vi "DataSocket-ImgSender.vi"() -> ()   [LabVIEW 2019]
doc: "Uses DataSocket to write array data. This example works for writing the data to the DataSocket Server (for live data). \n \nThe Writer, Server, and Reader can all be on the same computer or different computers. The Writer and Reader URLs should point to the computer where the DataSocket Server is."
panel:
  out "Image":T1(plugin-control)
  in  "Stop":bool
  # "DataSocket - Image Sender"
  # "Instruction:\n1. Run DataSocket Server;\n2. Run this VI;\n3. Run Image Receiver.\n4. see the images transfered\n to image reveiver."
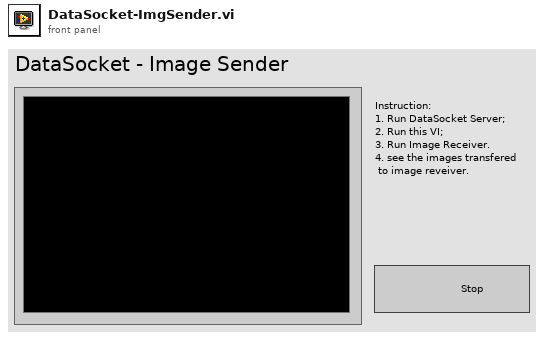
[diagram p1: front panel]
types:
  T1 = typedef "IMAQ Image.ctl" = refnum<image>
  T2 = enum16{"Read", "Write", "ReadWrite", "BufferedRead", "BufferedReadWrite"}
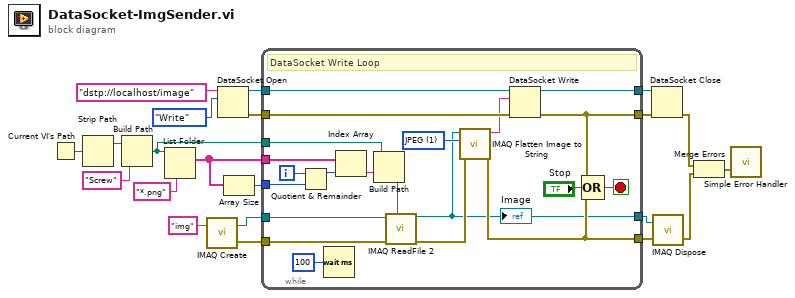
[diagram p0: block diagram]
diagram:
  n1 = Current VI's Path() -> (path=w12:path)
  n2 = Strip Path(path=w12) -> (stripped path=w11:path)  [unwired: 1 out]
  n3 = Build Path(base path=w11, name or relative path="Screw") -> (appended path=w6:path)
  n4 = List Folder(path=w6, pattern="*.png") -> (filenames=w4:string[])  [unwired: 2 in, 3 out]
  n5 = call "IMAQ Create"("Image Name"="img") -> ("New Image"=w7:T1, "error out"=w8:errorcluster)  [unwired: 4 in]
  n6 = DataSocket Open(10:T2."Write" ("mode"), 11:"dstp://localhost/image" ("Write Location")) -> (0:w19:errorcluster, 3:w20:refnum<k13>)  [unwired: 2 in]
  n7 = Array Size(array=w4) -> (size(s)=w5:i32)
  n8 = while {
    tunnel: [w26] -> w21
    tunnel: w20 -> [w39]
    tunnel: w19 -> [w38]
    tunnel: [w41] -> w18
    tunnel: [w24] -> w14
    tunnel: [w22] -> w13
    tunnel: w8 -> [w36]
    tunnel: w7 -> [w35]
    tunnel: w6 -> [w34]
    tunnel: w4 -> [w30]
    tunnel: w5 -> [w29]
    i -> [w31]
    stop <- w25 stop-if-true
    w40 = 1 items=["None", "JPEG", "PACKED BINARY"] ("Compression (None)")
    # "DataSocket Write Loop"
    n9 = Quotient & Remainder(x=w31, y=w29) -> (x-y*floor(x/y)=w32:i32)  [unwired: 1 out]
    n10 = Wait (ms)(milliseconds to wait=u32 100) -> ()  [unwired: 1 out]
    n11 = Index Array(array=w30, index=w32) -> (element=w28:string)
    n12 = Build Path(base path=w34, name or relative path=w28) -> (appended path=w33:path)
    n13 = call "IMAQ ReadFile 2"("File Path"=w33, "error in (no error)"=w36, "Image"=w35) -> ("error out"=w37:errorcluster, "Image Out"=w22:T1)  [unwired: 4 in, 3 out]
    "Image" <- w22
    n14 = call "IMAQ Flatten Image to String"("error in (no error)"=w37, "Compression (None)"=w40, "Image"=w22) -> ("error out"=w24:errorcluster, "Data String"=w27:string)  [unwired: 7 in]
    n15 = DataSocket Write(8:w38, 10:w27, 11:w39) -> (0:w26:errorcluster, 3:w41:refnum<k13>)  [unwired: 2 out]
    n16 = Compound Arithmetic op=OR(w26, "Stop", w24) -> (w25:bool)
  }
  n17 = DataSocket Close(8:w21, 11:w18) -> (0:w3:errorcluster)  [unwired: 1 in, 1 out]
  n18 = call "IMAQ Dispose"("Image"=w13, "error in (no error)"=w14) -> ("error out"=w2:errorcluster)  [unwired: 4 in]
  n19 = Merge Errors(w3, w2) -> (w1:errorcluster)
  n20 = call <vilib>:"Simple Error Handler.vi"("error in (no error)"=w1) -> ()  [unwired: 4 in, 5 out]
